vi "Split TDMS.vi"(7 "i":i32, 8 "error in":errorcluster, 9 "format string":string, 10 "split size (bytes)":i64, 11 "tdms file":refnum<k34>) -> (0 "error out":errorcluster, 3 "tdms file out":refnum<k34>, 5 "file changed":bool)   [LabVIEW 2010]
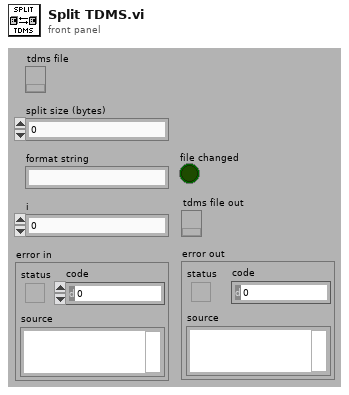
[diagram p1: front panel]
types:
  T1 = enum16{"open", "open or create", "create or replace", "create", "open (read-only)"}
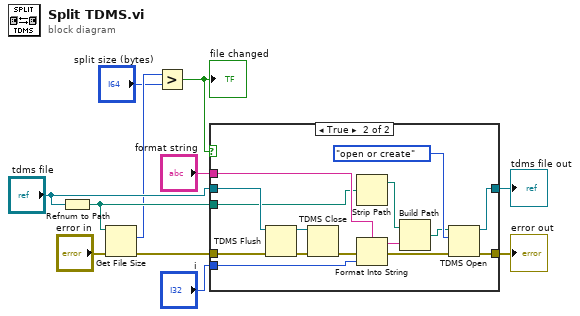
[diagram p0: block diagram]
diagram:
  n1 = Refnum to Path(1:"tdms file") -> (0:w5:path)
  n2 = Get File Size(file=w5, error in="error in") -> (size (in bytes)=w2:i64, 0:w9:errorcluster)  [unwired: 1 out]
  n3 = Greater?(x=w2, y="split size (bytes)") -> (0:w10:bool)
  "file changed" <- w10
  n4 = case shown="True" w10 {
    tunnel: "tdms file" -> [w12 w28]
    tunnel: w9 -> [w13 w24]
    tunnel: [w13 w23] -> w3
    tunnel: "format string" -> [_ w22]
    tunnel: "i" -> [_ w21]
    tunnel: [w12 w18] -> w4
    tunnel: w5 -> [_ w15]
    frame False {
    }
    frame True {
      n5 = TDMS Flush(4:w24, 7:w28) -> (0:w27:errorcluster, 3:w26:refnum<k34>)
      n6 = TDMS Close(8:w27, 11:w26) -> (0:w20:errorcluster)  [unwired: 1 out]
      n7 = Strip Path(path=w15) -> (stripped path=w14:path)  [unwired: 1 out]
      n8 = Format Into String(format string=w22, error in=w20, w21) -> (resulting string=w17:string, error out=w19:errorcluster)  [unwired: 1 in]
      n9 = Build Path(base path=w14, name or relative path=w17) -> (appended path=w16:path)
      n10 = TDMS Open(8:w19, 10:T1."open or create" ("operation (0:open)"), 11:w16) -> (0:w23:errorcluster, 3:w18:refnum<k34>)  [unwired: 3 in]
    }
  }
  "tdms file out" <- w4
  "error out" <- w3
